vi "escribe_tbl_igual_patrones.vi"(7 "last_id_ajuste_previo":string, 8 "error in (no error)":errorcluster, 9 "usuario_registra":i32=1, 10 "igualacion_de_patrones":T1, 11 "DB in":refnum<class "Base de Datos.lvclass">) -> (0 "error out":errorcluster, 3 "DB out":refnum<class "Base de Datos.lvclass">)   [LabVIEW 2019, in "Base de Datos.lvclass"]
uses:
  Base de Datos.lvclass
  Base de Datos.lvclass/Base de Datos.ctl
  SQLiteConnector/SQLiteConnection.lvclass
panel:
  out "Paso 2":string
  # "Tabla que registra los datos de la igualación de patrones 1"
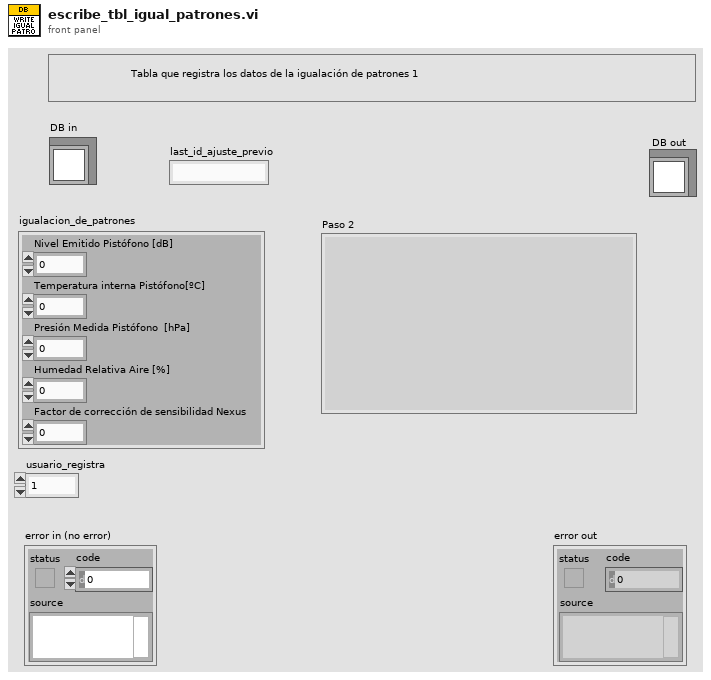
[diagram p1: front panel]
types:
  T1 = cluster{"Nivel Emitido Pistófono [dB]":dbl, "Temperatura interna Pistófono[ºC]":dbl, "Presión Medida Pistófono  [hPa]":dbl, "Humedad Relativa Aire [%]":dbl, "Factor de corrección de sensibilidad Nexus":dbl}
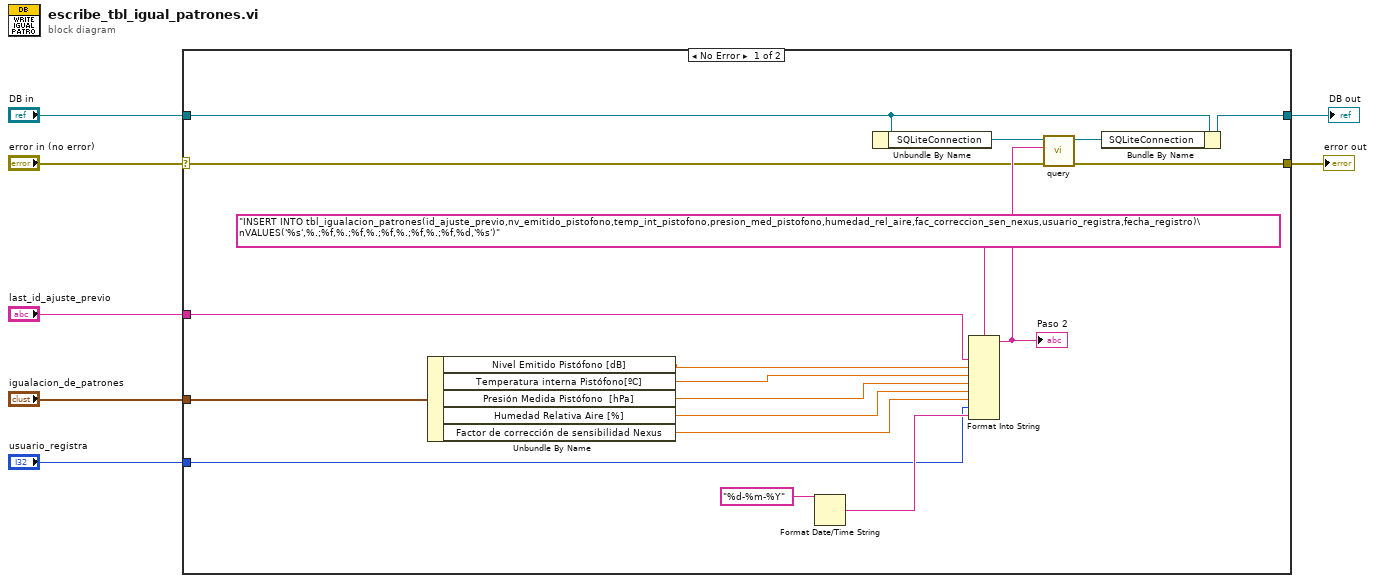
[diagram p0: block diagram]
diagram:
  n1 = case shown="No Error" "error in (no error)" {
    selector: "error in (no error)" -> [w14 w27]
    tunnel: [w25 w27] -> w7
    tunnel: "DB in" -> [w11 w26]
    tunnel: "igualacion_de_patrones" -> [w15 _]
    tunnel: "usuario_registra" -> [w13 _]
    tunnel: "last_id_ajuste_previo" -> [w12 _]
    tunnel: [w9 w26] -> w1
    frame No Error {
      n2 = Unbundle By Name(w15) -> ("Nivel Emitido Pistófono [dB]"=w20:dbl, "Temperatura interna Pistófono[ºC]"=w19:dbl, "Presión Medida Pistófono  [hPa]"=w18:dbl, "Humedad Relativa Aire [%]"=w17:dbl, "Factor de corrección de sensibilidad Nexus"=w16:dbl)
      n3 = Format Date/Time String(time format string (%c)="%d-%m-%Y") -> (date/time string=w21:string)  [unwired: 2 in]
      n4 = Unbundle By Name(w11) -> ("SQLiteConnection"=w10:refnum<class "SQLiteConnection.lvclass">)
      n5 = Format Into String(format string="INSERT INTO tbl_igualacion_patrones(id_ajuste_previo,nv_emitido_pistofono,temp_int_pistofono,presion_med_pistofono,humedad_rel_aire,fac_correccion_sen_nexus,usuario_registra,fecha_registro)\nVALUES('%s',%.;%f,%.;%f,%.;%f,%.;%f,%.;%f,%d,'%s')", w12, w20, w19, w18, w17, w16, w13, w21) -> (resulting string=w24:string)  [unwired: 2 in, 1 out]
      "Paso 2" <- w24
      n6 = call "query.vi"("error in (no error)"=w14, "SQL Statement"=w24, "object in"=w10) -> ("error out"=w25:errorcluster, "object out"=w8:refnum<class "SQLiteConnection.lvclass">)  [unwired: 5 in, 2 out]
      n7 = Bundle By Name(cluster=w11, "SQLiteConnection"=w8) -> (w9:refnum<class "Base de Datos.lvclass">)
    }
    frame Error {
    }
  }
  "error out" <- w7
  "DB out" <- w1
